vi "DialogManageInterfaces.vi"(8 "error in (no error)":errorcluster, 10 "ClassItemRefIn":refnum<vi>, 11 "ClassWriterIn":refnum<class "ClassWriter.lvclass">) -> (0 "error out":errorcluster, 1 "HandleInterfacesData":T1, 2 "Cancelled":bool, 3 "ClassWriterOut":refnum<class "ClassWriter.lvclass">)   [LabVIEW 2020, in "ClassWriter.lvclass"]
uses:
  ClassWriter.lvclass
  HandleInterfacesData.ctl
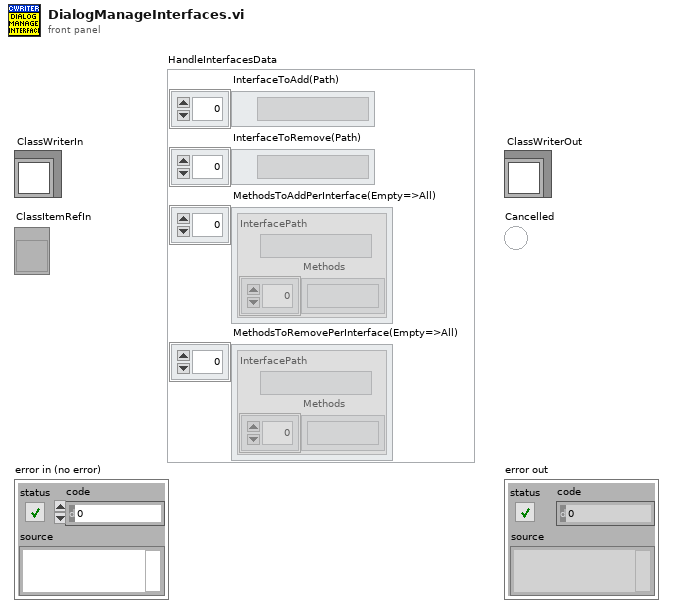
[diagram p1: front panel]
types:
  T1 = typedef "ClassWriter.lvclass/HandleInterfacesData.ctl" = cluster{"InterfaceToAdd(Path)":path[], "InterfaceToRemove(Path)":path[], "MethodsToAddPerInterface(Empty=>All)":cluster{"InterfacePath":path, "Methods":string[]}[], "MethodsToRemovePerInterface(Empty=>All)":cluster{"InterfacePath":path, "Methods":string[]}[]}
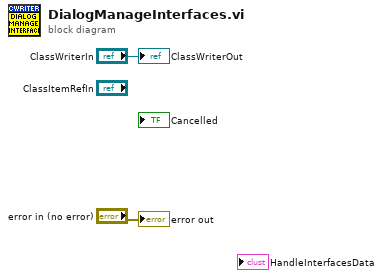
[diagram p0: block diagram]
diagram:
  "error out" <- "error in (no error)"
  "ClassWriterOut" <- "ClassWriterIn"
